vi "jl-scripts path.vi"() -> ()   [LabVIEW 2018, in "LV-0mq-Julia_roundtrip-lib.lvlib" / "LV2Julia_core.lvlib"]
uses:
  LV2Julia_core.lvlib
panel:
  out "jl-script file path":path
  out "tmp file path":path
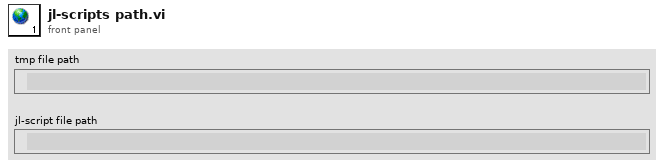
[diagram p1: front panel]
diagram:
